vi "Read Folder Shot File.vi"(8 "error in (no error)":errorcluster, 11 "Log Path":path) -> (0 "error out":errorcluster, 3 "Folder Shot":T1[](array[typedef]))   [LabVIEW 2016, in "SLL File IO.lvlib"]
doc: "Reads a Folder Shot file and returns the Folder Shot Cluster Array."
uses:
  SLL File IO.lvlib
  _Typedefs/Folder Shot Element.ctl
  <vilib>/Utility/file.llb/Read Delimited Spreadsheet (string).vi
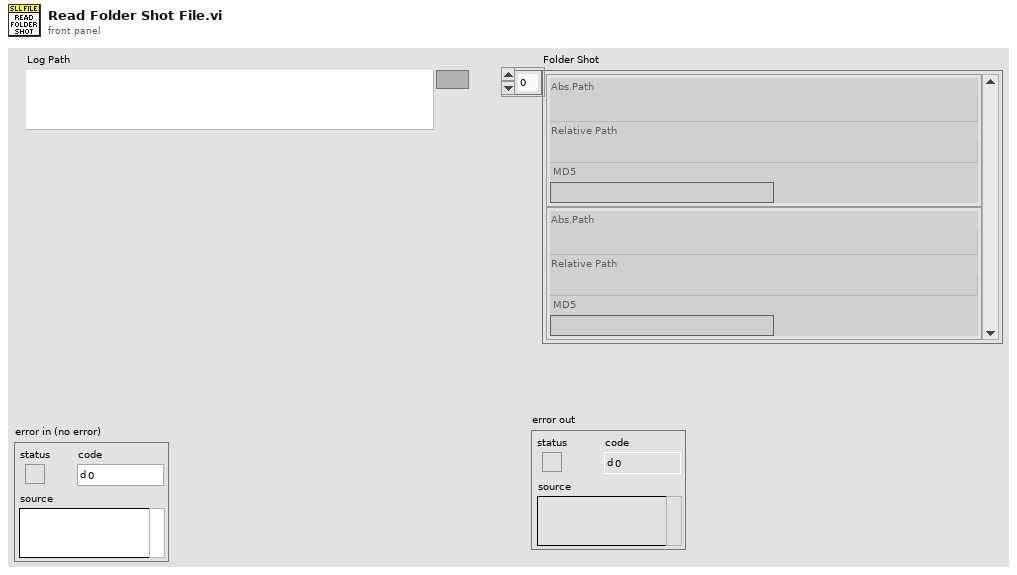
[diagram p1: front panel]
types:
  T1 = typedef "SLL File IO.lvlib/Folder Shot Element.ctl" = cluster{"Abs.Path":path, "Relative Path":path, "MD5":string}
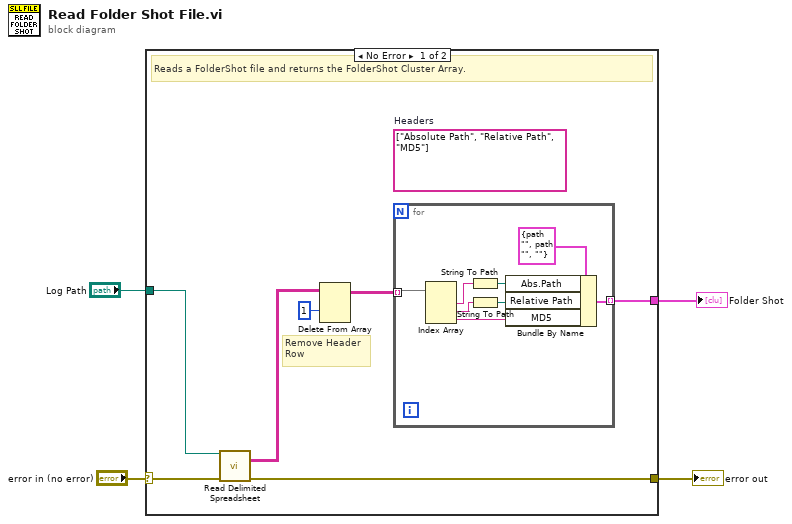
[diagram p0: block diagram]
diagram:
  n1 = case shown="No Error" "error in (no error)" {
    selector: "error in (no error)" -> [w6 w20]
    tunnel: [w7 w20] -> w3
    tunnel: "Log Path" -> [w11 _]
    tunnel: [w8 _] -> w1
    frame No Error {
      (unwired) string[] ["Absolute Path", "Relative Path", "MD5"]  # Headers
      # "Remove Header\nRow"
      # "Reads a FolderShot file and returns the FolderShot Cluster Array."
      n2 = call-poly <vilib>:"Read Delimited Spreadsheet.vi"("file path (dialog if empty)"=w11, "error in (no error)"=w6) -> ("all rows"=w5:string[][], "error out"=w7:errorcluster)  [unwired: 8 in, 4 out]
      n3 = Delete From Array(array=w5, index (row)=1) -> (array with subset deleted=w9:string[][])  [unwired: 2 in, 1 out]
      n4 = for {
        tunnel: w9 -> [w19] mode=indexing
        tunnel: [w12] -> w8 mode=indexing
        n5 = Index Array(array=w19) -> (element #1=w16:string, element #2=w14:string, element #3=w17:string)  [unwired: 3 in]
        n6 = String To Path(string=w16) -> (path=w15:path)
        n7 = String To Path(string=w14) -> (path=w13:path)
        n8 = Bundle By Name(cluster=T1 {"Abs.Path"=path "", "Relative Path"=path "", "MD5"=""} ("Folder Shot Element"), "Abs.Path"=w15, "Relative Path"=w13, "MD5"=w17) -> (w12:T1)
      }
    }
    frame Error {
    }
  }
  "error out" <- w3
  "Folder Shot" <- w1
